vi "CRYGet Global RcvBuffer.vi"(6 "bufCount In":i32, 9 "Chn Idx":u32) -> (0 "bufCount":i32, 1 "rtn value":i32, 3 "Data":i32[](array[numeric]))   [LabVIEW 2013]
uses:
  CRYMisc vis settings global.vi
panel:
  out "size(s)":i32
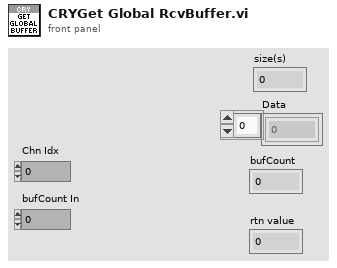
[diagram p1: front panel]
types:
  T1 = cluster{"Rcv Idx":i32, "Chn Idx":i32, "Data":i32[], "bufCount":i32}[]
  T2 = cluster{"Rcv Idx":i32, "Chn Idx":i32, "Data":i32[], "bufCount":i32}
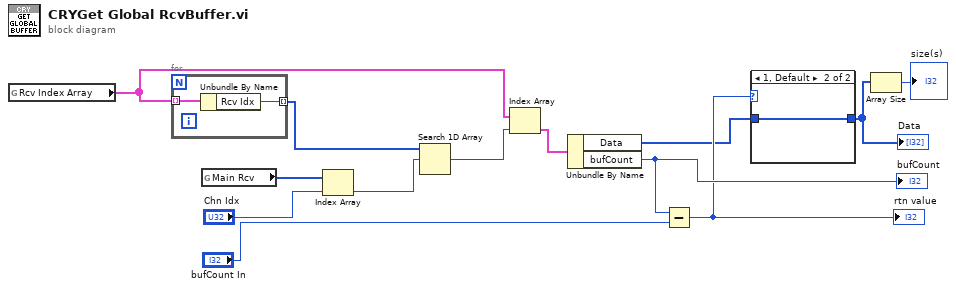
[diagram p0: block diagram]
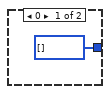
[diagram p2: hidden frame]
diagram:
  n1 = global read "CRYMisc vis settings global.vi" "Rcv Index Array"() -> (w9:T1)
  n2 = for {
    tunnel: w9 -> [w15] mode=indexing
    tunnel: [w14] -> w11 mode=indexing
    n3 = Unbundle By Name(w15) -> ("Rcv Idx"=w14:i32)
  }
  n4 = global read "CRYMisc vis settings global.vi" "Main Rcv"() -> (w13:i32[])
  n5 = Index Array(array=w13, index="Chn Idx") -> (element=w10:i32)
  n6 = Search 1D Array(1D array=w11, element=w10) -> (index of element=w8:i32)  [unwired: 1 in]
  n7 = Index Array(array=w9, index=w8) -> (element=w7:T2)
  n8 = Unbundle By Name(w7) -> ("Data"=w3:i32[], "bufCount"=w6:i32)
  "bufCount" <- w6
  n9 = Subtract(x=w6, y="bufCount In") -> (x-y=w4:i32)
  "rtn value" <- w4
  n10 = case shown="1, Default" w4 {
    tunnel: w3 -> [_ w17]
    tunnel: [i32[] [] ("Data") w17] -> w2
    frame 0 {
    }
    frame 1, Default {
    }
  }
  "Data" <- w2
  n11 = Array Size(array=w2) -> (size(s)=→"size(s)":i32)
